vi "MainNR.vi"(10 "JQMHStartup":refnum<class "ModuleStartup.lvclass">, 11 "ErrorViewer in":refnum<class "ErrorViewer.lvclass">) -> ()   [LabVIEW 2025, in "ErrorViewer.lvclass"]
uses:
  ErrorViewer.lvclass
  C:/Git/JA/JQMH/RQMHCore/ModuleCore/Module.lvclass
  RQMHCore/Startup/ModuleStartup.lvclass
  RQMHCore/ErrorReporting/Record/LogRecord.lvclass
  RQMHCore/ModuleCore/Module.lvclass/Module.ctl
  RQMHCore/ErrorReporting/Record/LogRecord.lvclass/LogRecord.ctl
  ErrorLogBuffer/ErrorLogBuffer.lvclass/ErrorLogBuffer.ctl
  RQMHCore/ModuleCore/Reply.ctl
  RQMHCore/ActionStack/Stack/Stack.lvclass/Stack.ctl
  RQMHCore/ModuleCore/InitialiseReplyArgs.ctl
  <vilib>/Utility/miscctls.llb/LVPointTypeDef.ctl
  <vilib>/Utility/miscctls.llb/LVRowAndColumnTypeDef.ctl
  Do Something ReplyArgs.ctl
  RQMHCore/ErrorReporting/Record/Read Time.vi
  RQMHCore/ErrorReporting/Record/Read Level.vi
  RQMHCore/ErrorReporting/Record/Read Source.vi
  RQMHCore/ErrorReporting/Record/Read Message.vi
  RQMHCore/ActionStack/Stack/AppendStacks.vi
  RQMHCore/ModuleCore/Read ModuleName.vi
  RQMHCore/ErrorReporting/Record/Read Error.vi
  ErrorLogBuffer/Wrap.vi
  RQMHCore/ActionStack/Stack/StackFromSingleWithPayload.vi
  RQMHCore/ActionStack/Stack/InitFromString.vi
  RQMHCore/ActionStack/Stack/Stack.lvclass
  RQMHCore/ModuleCore/Module.lvclass
  DataStructures/src/DataTypes/Cyclic Table/Cyclic Table.lvclass
  ErrorLogBuffer/ErrorLogBuffer.lvclass
panel:
  out "Error":errorcluster
  out "error out":errorcluster
  out "Table":string[][](table)
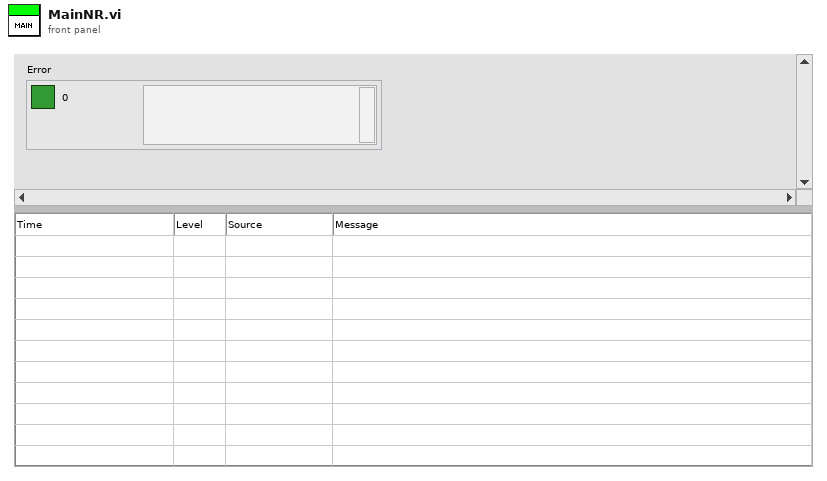
[diagram p1: front panel]
types:
  T1 = typedef "ErrorViewer.lvclass/Request Events--cluster.ctl" = cluster{"Do Something":refnum<user-event>, "Inject Log Event":refnum<user-event>}
  T2 = cluster{"StandardRequests":refnum<event-registration>, "Event Registration Refnum":refnum<event-registration>}
  T3 = cluster{"Module":refnum<class "ErrorViewer.lvclass">, "ErrorLog":refnum<class "ErrorLogBuffer.lvclass">, "Cyclic Table":refnum<class "Cyclic Table.lvclass">}
  T4 = typedef "Module.lvclass/Reply.ctl" = cluster{"Expects Reply":bool, "Reply":refnum<notifier>}
  T5 = enum32{"Invalid", "Standard", "Closed", "Hidden", "Minimized", "Maximized"}
  T6 = typedef "Module.lvclass/InitialiseReplyArgs.ctl" = cluster{"Did Init?":bool}
  T7 = typedef "LVPointTypeDef.ctl" = cluster{"Horizontal":i16, "Vertical":i16}
  T8 = typedef "LVRowAndColumnTypeDef.ctl" = cluster{"Row":i32, "Column":i32}
  T9 = typedef "ErrorViewer.lvclass/Do Something ReplyArgs.ctl" = cluster{"Value":dbl}
  T10 = typedef "JQMHModule.lvclass/Show Front Panel--Args.ctl" = variant
  T11 = typedef "JQMHModule.lvclass/Show Block Diagram.ctl" = bool
  T12 = typedef "JQMHModule.lvclass/Reply.ctl" = cluster{"Expects Reply":bool, "Reply":refnum<notifier>}
  T13 = typedef "LVPoint32TypeDef.ctl" = cluster{"Horizontal":i32, "Vertical":i32}
  T14 = typedef "LoggerShared.lvlib/Level.ctl" = enum16{"DEBUG", "INFO", "WARNING", "ERROR", "CRITICAL"}
  T15 = typedef "ErrorViewer.lvclass/Do Something Args.ctl" = cluster{"Msg":string}
  T16 = typedef "ErrorLogBuffer.lvclass/Type.ctl" = refnum<class "LogRecord.lvclass">
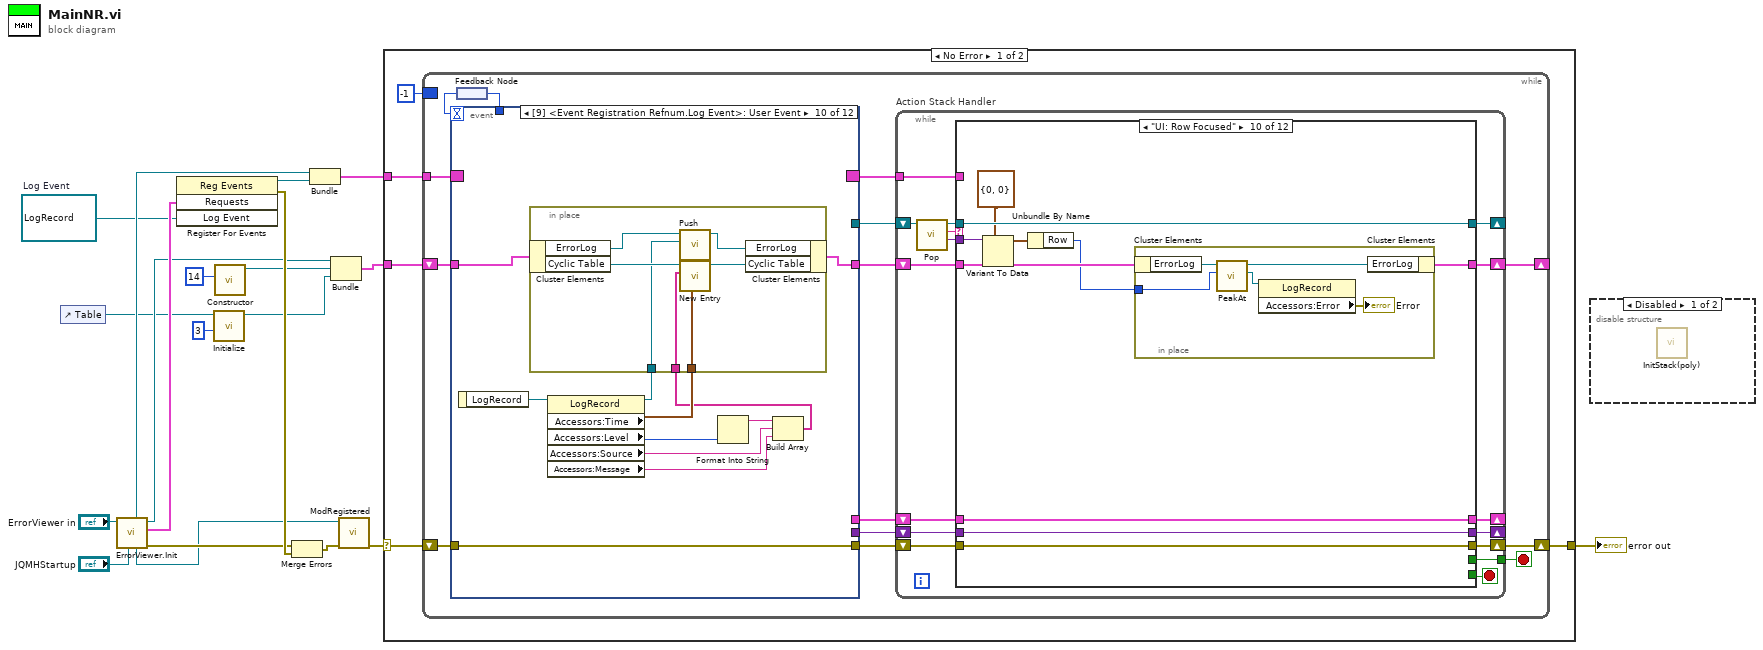
[diagram p0: block diagram]
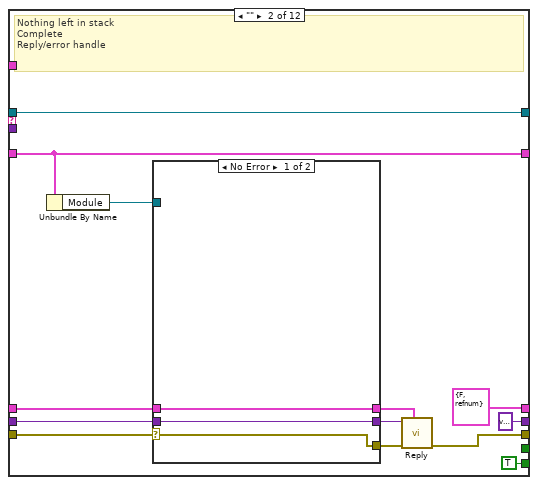
[diagram p3: hidden frame]
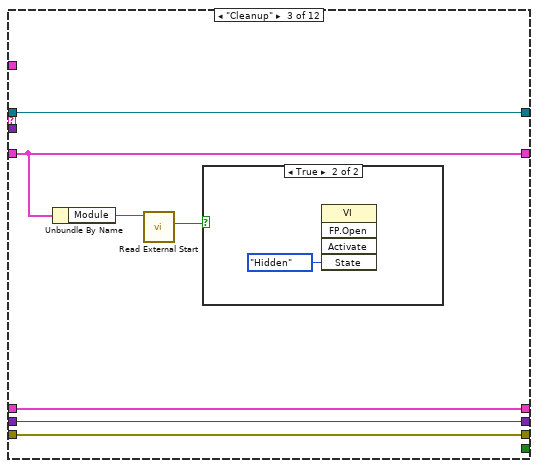
[diagram p5: hidden frame]
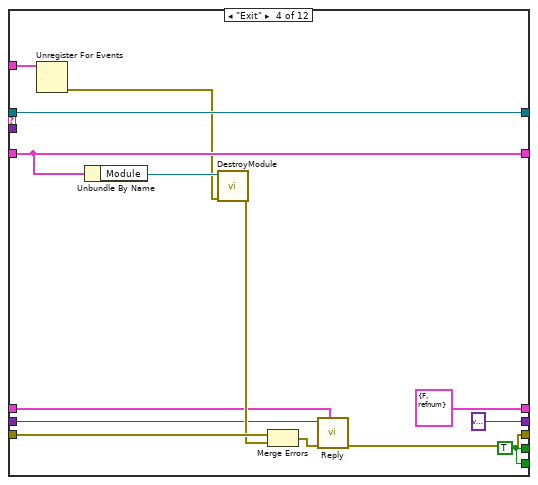
[diagram p7: hidden frame]
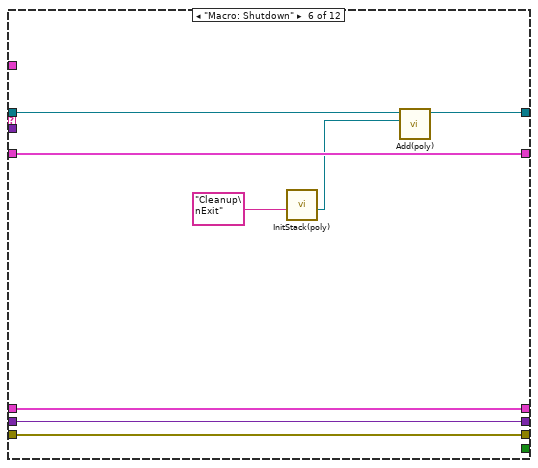
[diagram p9: hidden frame]
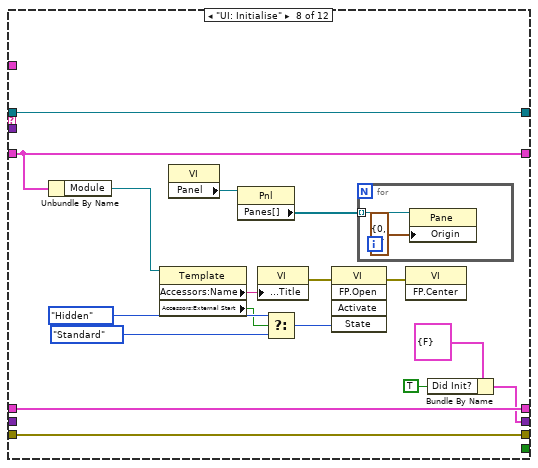
[diagram p11: hidden frame]
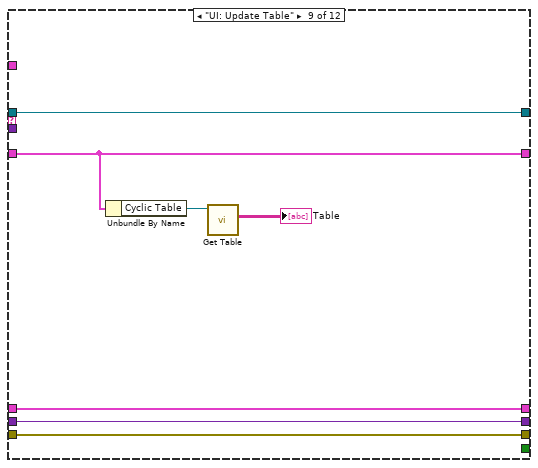
[diagram p12: hidden frame]
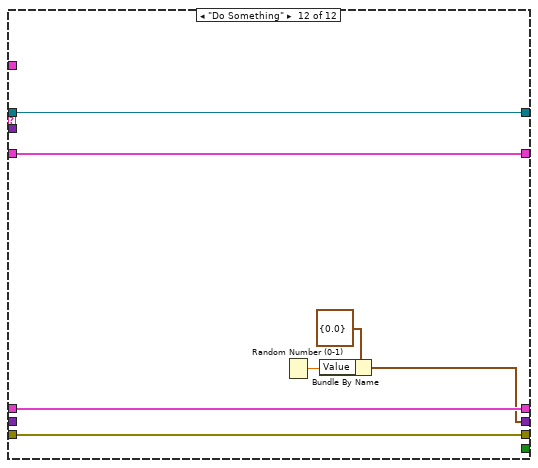
[diagram p14: hidden frame]
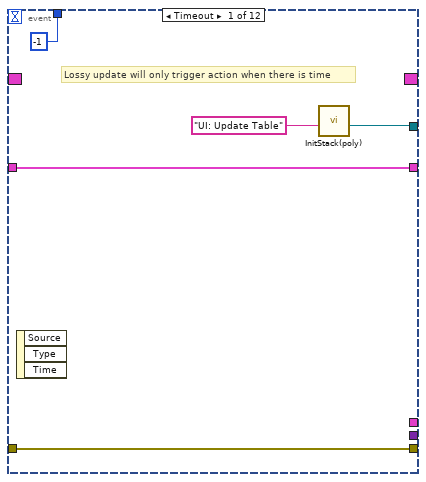
[diagram p15: hidden frame]
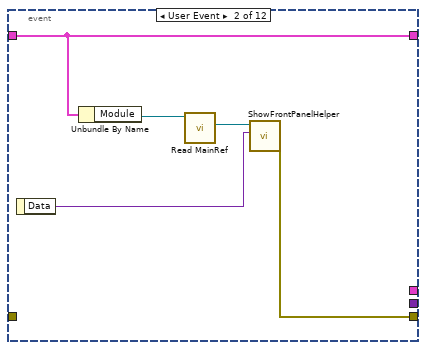
[diagram p16: hidden frame]
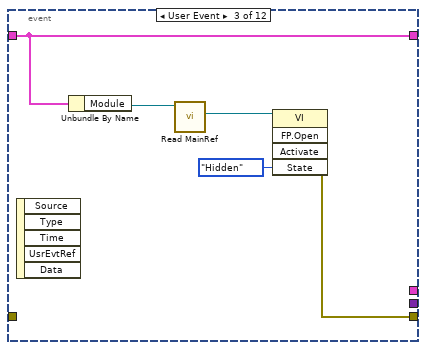
[diagram p17: hidden frame]
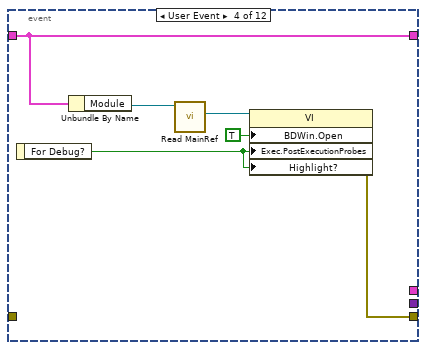
[diagram p18: hidden frame]
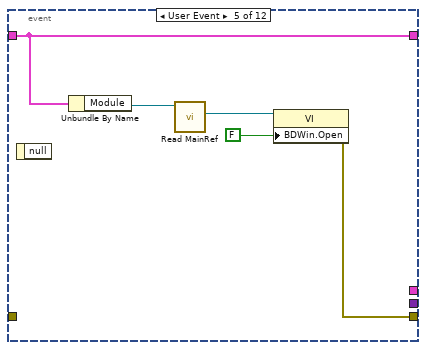
[diagram p19: hidden frame]
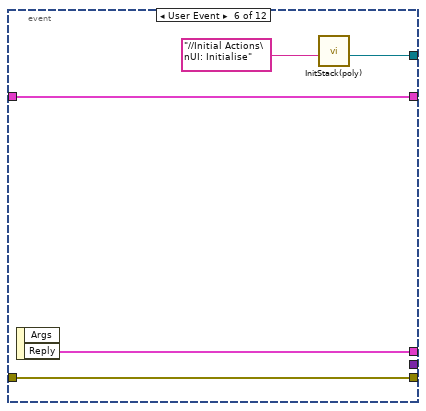
[diagram p20: hidden frame]
diagram:
  w6 = refnum<user-event> refnum  # Log Event
  n1 = control-ref of="Table"() -> (w4:refnum<vi>)
  n2 = call "ErrorViewer.Init.vi"("JQMHStartup in"="JQMHStartup", "ErrorViewer in"="ErrorViewer in") -> ("error out"=w16:errorcluster, "Requests"=w11:T1, "Module"=w8:refnum<class "ErrorViewer.lvclass">, "JQMHStartup out"=w15:refnum<class "ModuleStartup.lvclass">, "StandardRequests"=w7:refnum<event-registration>)  [unwired: 3 in, 2 out]
  n3 = register-events(w11, w6) -> (reference out=w12:refnum<event-registration>, error out=w20:errorcluster)  [unwired: 2 in]
  n4 = call "Initialize.vi"("# columns"=3, "Table"=w4) -> ("Cyclic Table"=w5:refnum<class "Cyclic Table.lvclass">)  [unwired: 8 in, 1 out]
  n5 = call "Constructor.vi"("Capacity 2^n"=u32 14 ("Capacity")) -> ("ErrorLog"=w2:refnum<class "ErrorLogBuffer.lvclass">)  [unwired: 10 in]
  n6 = Merge Errors(w16, w20) -> (w13:errorcluster)
  n7 = Bundle("StandardRequests"=w7, "Event Registration Refnum"=w12) -> (w9:T2)  [unwired: 1 in]
  n8 = Bundle("Module"=w8, "ErrorLog"=w2, "Cyclic Table"=w5) -> (w10:T3)  [unwired: 1 in]
  n9 = call "ModRegistered.vi"("error in (no error)"=w13, "JQMHStartup in"=w15) -> ("error out"=w14:errorcluster)  [unwired: 9 in]
  n10 = case "RQMH_MAIN" shown="No Error" w14 {
    selector: w14 -> [w24 w259]
    tunnel: w9 -> [w22 w258]
    tunnel: [w25 w259] -> w18
    tunnel: w10 -> [w23 w257]
    frame No Error {
      n11 = while {
        shift-right: [w32] -> w25
        shift-left: w24 -> [w39]
        shift-right: [w34] -> _
        shift-left: w23 -> [w35]
        tunnel: w22 -> [w28]
        border: -1 -> [_]
        stop <- w31 stop-if-true
        n12 = feedback #1() -> (w26:i32)
        n13 = event "RQMH_EVENT_MAIN" shown="[9] <Event Registration Refnum.Log Event>: User Event" {
          selector: w28 -> [_ _ _ _ _ _ _ _ _ _ _ w254]
          dyn-events: [_ _ _ _ _ _ _ _ _ _ _ _] -> w38
          timeout: w26 -> [_ _ _ _ _ _ _ _ _ _ _ _]
          tunnel: w39 -> [w177 _ _ _ _ w203 w208 w217 w224 w235 w248 w250]
          tunnel: [w177 w179 w183 w188 w194 w203 w208 w217 w224 w235 w248 w252] -> w33
          tunnel: [w173 _ _ _ _ w199 w204 w215 w218 _ w243 _] -> w37
          tunnel: w35 -> [w176 w182 w185 w192 w197 w202 w206 w214 w223 w233 w246 w255]
          tunnel: [w176 w182 w185 w192 w197 w202 w206 w214 w223 w234 w246 w255] -> w36
          tunnel: [_ _ _ _ _ w201 _ _ _ _ w244 w249] -> w30
          tunnel: [_ _ _ _ _ _ variant _ _ _ _ _] -> w29
          tunnel: [-1 _ _ _ _ _ _ _ _ _ _ _] -> w27
          event Timeout {
            # "Lossy update will only trigger action when there is time"
            n14 = event-data() -> ()  [unwired: 1 in, 3 out]
            n15 = call-poly "InitStack(poly).vi"("Action"="UI: Update Table") -> ("Stack out"=w173:refnum<class "Stack.lvclass">)  [unwired: 10 in]
          }
          event User Event {
            n16 = event-data() -> ("Data"=w178:T10)  [unwired: 1 in]
            n17 = Unbundle By Name(w182) -> ("Module"=w181:refnum<class "ErrorViewer.lvclass">)
            n18 = call "Read MainRef.vi"("RQMHModule in"=w181) -> ("MainRef"=w180:refnum<vi>)  [unwired: 8 in, 2 out]
            n19 = call "ShowFrontPanelHelper.vi"("Data"=w178, "VI in"=w180) -> ("error out"=w179:errorcluster)  [unwired: 9 in]
          }
          event User Event {
            n20 = event-data() -> ()  [unwired: 1 in, 5 out]
            n21 = Unbundle By Name(w185) -> ("Module"=w186:refnum<class "ErrorViewer.lvclass">)
            n22 = call "Read MainRef.vi"("RQMHModule in"=w186) -> ("MainRef"=w184:refnum<vi>)  [unwired: 8 in, 2 out]
            n23 = invoke class="VI" method="FP.Open"(reference=w184, "State"=T5."Hidden") -> (error out=w183:errorcluster)  [unwired: 3 in, 4 out]
          }
          event User Event {
            n24 = event-data() -> ("For Debug?"=w189:T11)  [unwired: 1 in]
            n25 = Unbundle By Name(w192) -> ("Module"=w193:refnum<class "ErrorViewer.lvclass">)
            n26 = call "Read MainRef.vi"("RQMHModule in"=w193) -> ("MainRef"=w190:refnum<vi>)  [unwired: 8 in, 2 out]
            n27 = property class="VI"(reference=w190, "BDWin.Open"=TRUE ("Block Diagram Window:Open"), "Exec.PostExecutionProbes"=w189, "Highlight?"=w189) -> (error out=w188:errorcluster)  [unwired: 1 in, 1 out]
          }
          event User Event {
            n28 = event-data() -> ()  [unwired: 1 in, 1 out]
            n29 = Unbundle By Name(w197) -> ("Module"=w198:refnum<class "ErrorViewer.lvclass">)
            n30 = call "Read MainRef.vi"("RQMHModule in"=w198) -> ("MainRef"=w195:refnum<vi>)  [unwired: 8 in, 2 out]
            n31 = property class="VI"(reference=w195, "BDWin.Open"=FALSE ("Block Diagram Window:Open")) -> (error out=w194:errorcluster)  [unwired: 1 in, 1 out]
          }
          event User Event {
            n32 = event-data() -> ("Reply"=w201:T12)  [unwired: 1 in, 1 out]
            n33 = call-poly "InitStack(poly).vi"("ActionStack String"="//Initial Actions\nUI: Initialise") -> ("ActionStack out"=w199:refnum<class "Stack.lvclass">)  [unwired: 10 in]
          }
          event User Event {
            (unwired) errorcluster {"status"=FALSE, "code"=0, "source"=""} ("error out")
            (unwired) TRUE
            n34 = event-data() -> ()  [unwired: 1 in, 1 out]
            n35 = call-poly "InitStack(poly).vi"("Action"="Macro: Shutdown") -> ("Stack out"=w204:refnum<class "Stack.lvclass">)  [unwired: 10 in]
          }
          event Panel Close? {
            n36 = event-data() -> ()  [unwired: 1 in, 4 out]
            n37 = Unbundle By Name(w214) -> ("Module"=w213:refnum<class "ErrorViewer.lvclass">)
            n38 = call "Read External Start.vi"("JQMHModule in"=w213) -> ("External Start?"=w212:bool)  [unwired: 8 in, 2 out]
            n39 = Select(t="", s=w212, f="Macro: Shutdown" ("Action")) -> (s? t:f=w209:string)
            n40 = call-poly "InitStack(poly).vi"("Action"=w209) -> ("Stack out"=w215:refnum<class "Stack.lvclass">)  [unwired: 10 in]
            n41 = event-data("Discard?"=TRUE) -> ()  [unwired: 1 in, 1 out]
          }
          event "Table": Mouse Down? {
            n42 = event-data() -> ("CtlRef"=w222:refnum<vi>, "Coords"=w221:T13)  [unwired: 1 in, 1 out]
            n43 = invoke class="Tbl (strict)" method="Point To Row Column"(reference=w222, "Point"=w221) -> ("CellPosition"=w219:T8)  [unwired: 4 in, 5 out]
            n44 = event-data() -> ()  [unwired: 5 in, 1 out]
            n45 = call-poly "InitStack(poly).vi"("Payload"=w219, "Action"="UI: Row Focused") -> ("Stack out"=w218:refnum<class "Stack.lvclass">)  [unwired: 9 in]
          }
          event User Event {
            n46 = event-data() -> ("LogRecord"=w232:refnum<class "LogRecord.lvclass">)  [unwired: 1 in]
            n47 = property class="LogRecord"(reference=w232) -> (reference out=w225:refnum<class "LogRecord.lvclass">, "Accessors:Time"=w231:timestamp, "Accessors:Level"=w230:T14, "Accessors:Source"=w228:string, "Accessors:Message"=w227:string)  [unwired: 1 in, 1 out]
            n48 = Format Into String(w230) -> (resulting string=w229:string)  [unwired: 3 in, 1 out]
            n49 = Build Array(w229, w228, w227) -> (w226:string[])
            n50 = in-place {
              in-place-border: w231 -> [w240]
              in-place-border: w226 -> [w239]
              in-place-border: w225 -> [w236]
              n51 = in-place-cluster #2(w233) -> ("ErrorLog"=w238:refnum<class "ErrorLogBuffer.lvclass">, "Cyclic Table"=w242:refnum<class "Cyclic Table.lvclass">)
              n52 = call "Push.vi"("Element"=w236, "POTTypedCircularBuffer in"=w238) -> ("POTTypedCircularBuffer in"=w237:refnum<class "ErrorLogBuffer.lvclass">)  [unwired: 9 in]
              n53 = call "New Entry.vi"("Time Stamp (Now)"=w240, "New Entry"=w239, "Cyclic Table in"=w242) -> ("Cyclic Table out"=w241:refnum<class "Cyclic Table.lvclass">)  [unwired: 8 in]
              n54 = in-place-cluster #2("ErrorLog"=w237, "Cyclic Table"=w241) -> (w234:T3)
            }
          }
          event User Event {
            n55 = event-data() -> ("Args"=w245:T15, "Reply Payload"=w244:T4)  [unwired: 1 in]
            n56 = call-poly "InitStack(poly).vi"("Payload"=w245, "Action"="Do Something" ("Message")) -> ("Stack out"=w243:refnum<class "Stack.lvclass">)  [unwired: 9 in]
          }
          event User Event {
            n57 = event-data() -> ("Args.Log Event"=w251:refnum<user-event>, "Reply Payload"=w249:T4)  [unwired: 1 in]
            n58 = Unbundle By Name(w254) -> ("Event Registration Refnum"=w253:refnum<event-registration>)
            n59 = register-events(reference=w253, error in=w250, w251) -> (error out=w252:errorcluster)  [unwired: 1 in, 1 out]
          }
        }
        n60 = feedback-in #1(w27) -> ()
        n61 = while "Action Stack Handler" {
          shift-right: [w55] -> _
          shift-left: w37 -> [w47]
          shift-right: [w52] -> w32
          shift-left: w33 -> [w53]
          tunnel: w38 -> [w51]
          shift-right: [w49] -> w34
          shift-left: w36 -> [w50]
          tunnel: [w48] -> w31
          shift-right: [w42] -> _
          shift-left: w30 -> [w43]
          shift-right: [w41] -> _
          shift-left: w29 -> [w40]
          stop <- w54 stop-if-true
          n62 = call "Pop.vi"("Stack in"=w47) -> ("Popped Payload"=w44:variant, "Popped Action"=w45:string, "Stack out"=w46:refnum<class "Stack.lvclass">)  [unwired: 8 in]
          n63 = case shown="\"UI: Row Focused\"" w45 {
            tunnel: w46 -> [w60 w73 w86 w101 w106 w109 w119 w136 w145 w155 w165 w172]
            tunnel: [w60 w73 w86 w101 w106 w107 w119 w136 w145 w155 w165 w172] -> w55
            tunnel: w44 -> [_ _ _ _ _ _ _ _ _ w151 _ _]
            tunnel: [_ TRUE ("Boolean") _ w99 _ _ _ _ _ _ _ _] -> w54
            tunnel: w53 -> [w56 w71 w85 w93 w104 w113 w118 w135 w144 w154 w164 w171]
            tunnel: [w56 w66 w85 w88 w104 w113 w118 w135 w144 w154 w164 w171] -> w52
            tunnel: w51 -> [_ _ _ w100 _ _ _ _ _ _ _ _]
            tunnel: w50 -> [w59 w70 w81 w95 w105 w114 w117 w128 w141 w148 w163 w170]
            tunnel: [w59 w70 w81 w95 w105 w114 w117 w128 w141 w146 w163 w170] -> w49
            tunnel: [_ _ _ w99 _ _ _ _ _ _ _ _] -> w48
            tunnel: w43 -> [w58 w67 w84 w89 w103 w112 w116 w134 w143 w153 w162 w169]
            tunnel: [w58 T4 {"Expects Reply"=FALSE, "Reply"=refnum} ("Reply Payload") w84 T4 {"Expects Reply"=FALSE, "Reply"=refnum} ("Reply Payload") w103 w112 w116 w134 w143 w153 w162 w169] -> w42
            tunnel: [w57 variant ("Variant") w83 variant ("Variant") w102 w111 w115 w120 w142 w152 w161 w166] -> w41
            tunnel: w40 -> [w57 w62 w83 w90 w102 w111 w115 _ w142 w152 w161 _]
            frame Default {
              # "#TODO Add Error Handling"
            }
            frame "" {
              # "Nothing left in stack\nComplete\nReply/error handle"
              n64 = Unbundle By Name(w70) -> ("Module"=w69:refnum<class "ErrorViewer.lvclass">)
              n65 = case shown="No Error" w71 {
                selector: w71 -> [w74 w78]
                tunnel: [w76 w79] -> w68
                tunnel: w67 -> [w76 w79]
                tunnel: [w75 w77] -> w63
                tunnel: w62 -> [w75 w77]
                tunnel: w69 -> [_ _]
                tunnel: [w74 w78] -> w61
                frame No Error {
                }
                frame Error {
                }
              }
              n66 = call "Reply.vi"("Reply"=w68, "error in (no error)"=w61, "ReplyPayload"=w63) -> ("error out"=w66:errorcluster)  [unwired: 8 in]
            }
            frame "Cleanup" {
              n67 = Unbundle By Name(w81) -> ("Module"=w82:refnum<class "ErrorViewer.lvclass">)
              n68 = call "Read External Start.vi"("JQMHModule in"=w82) -> ("External Start?"=w80:bool)  [unwired: 8 in, 2 out]
              n69 = case shown="True" w80 {
                frame False {
                }
                frame True {
                  n70 = invoke class="VI" method="FP.Open"("State"=T5."Hidden") -> ()  [unwired: 4 in, 5 out]
                }
              }
            }
            frame "Exit" {
              w99 = TRUE
              n71 = Unregister For Events(event registration refnum=w100) -> (error out=w94:errorcluster)  [unwired: 1 in]
              n72 = Unbundle By Name(w95) -> ("Module"=w96:refnum<class "ErrorViewer.lvclass">)
              n73 = call "DestroyModule.vi"("error in (no error)"=w94, "JQMHModule in"=w96) -> ("error out"=w92:errorcluster)  [unwired: 9 in]
              n74 = Merge Errors(w93, w92) -> (w91:errorcluster)
              n75 = call "Reply.vi"("Reply"=w89, "error in (no error)"=w91, "ReplyPayload"=w90) -> ("error out"=w88:errorcluster)  [unwired: 8 in]
            }
            frame "---------- Macros ----------" {
            }
            frame "Macro: Shutdown" {
              n76 = call-poly "InitStack(poly).vi"("ActionStack String"="Cleanup\nExit") -> ("ActionStack out"=w108:refnum<class "Stack.lvclass">)  [unwired: 10 in]
              n77 = call-poly "Add(poly).vi"("Second"=w108, "First"=w109) -> ("First"=w107:refnum<class "Stack.lvclass">)  [unwired: 9 in]
            }
            frame "---------- UI ----------" {
              # "Add module specific commands"
            }
            frame "UI: Initialise" {
              n78 = Unbundle By Name(w128) -> ("Module"=w127:refnum<class "ErrorViewer.lvclass">)
              n79 = property class="Template"(reference=w127) -> ("Accessors:Name"=w126:string, "Accessors:External Start"=w124:bool)  [unwired: 1 in, 2 out]
              n80 = property on="Property Node" class="VI"() -> ("Panel"=w130:refnum<vi>)  [unwired: 2 in, 2 out]
              n81 = property on="Property Node" class="Pnl"(reference=w130) -> ("Panes[]"=w129:refnum<vi>[])  [unwired: 1 in, 2 out]
              n82 = property on="Property Node" class="VI"("Front Panel.Title"=w126) -> (error out=w133:errorcluster)  [unwired: 2 in, 1 out]
              n83 = Select(t=T5."Hidden" ("State"), s=w124, f=T5."Standard" ("State")) -> (s? t:f=w123:T5)
              n84 = invoke on="Invoke Node" class="VI" method="FP.Open"(error in=w133, "State"=w123) -> (error out=w132:errorcluster)  [unwired: 3 in, 4 out]
              n85 = for {
                tunnel: w129 -> [w137] mode=indexing
                n86 = property on="Property Node" class="Pane"(reference=w137, "Origin"=T7 {"Horizontal"=0, "Vertical"=0}) -> ()  [unwired: 1 in, 2 out]
              }
              n87 = invoke on="Invoke Node" class="VI" method="FP.Center"(error in=w132) -> ()  [unwired: 2 in, 3 out]
              n88 = Bundle By Name(cluster=T6 {"Did Init?"=FALSE} ("Args"), "Did Init?"=TRUE) -> (w120:T6)
            }
            frame "UI: Update Table" {
              n89 = Unbundle By Name(w141) -> ("Cyclic Table"=w140:refnum<class "Cyclic Table.lvclass">)
              n90 = call "Get Table.vi"("Cyclic Table in"=w140) -> ("Table Data (sorted by time)"=→"Table":string[][])  [unwired: 10 in]
            }
            frame "UI: Row Focused" {
              n91 = Variant To Data(type=T8 {"Row"=0, "Column"=0} ("Cell Position"), Variant=w151) -> (data=w149:T8)  [unwired: 1 in, 1 out]
              n92 = Unbundle By Name(w149) -> ("Row"=w147:i32)
              n93 = in-place {
                in-place-border: w147 -> [w156]
                n94 = in-place-cluster #3(w148) -> ("ErrorLog"=w160:refnum<class "ErrorLogBuffer.lvclass">)
                n95 = call "PeakAt.vi"("Index"=w156, "POTTypedCircularBuffer in"=w160) -> ("element"=w158:T16, "POTTypedCircularBuffer out"=w159:refnum<class "ErrorLogBuffer.lvclass">)  [unwired: 8 in]
                n96 = property class="LogRecord"(reference=w158) -> ("Accessors:Error"=→"Error":errorcluster)  [unwired: 1 in, 2 out]
                n97 = in-place-cluster #3("ErrorLog"=w159) -> (w146:T3)
              }
            }
            frame "---------- Actions ----------" {
              # "Add module specific commands"
            }
            frame "Do Something" {
              n98 = Random Number (0-1)() -> (number: 0 to 1=w168:dbl)
              n99 = Bundle By Name(cluster=T9 {"Value"=0.0} ("ReplyArgs"), "Value"=w168) -> (w166:T9)
            }
          }
        }
      }
    }
    frame Error {
      n100 = Unregister For Events(event registration refnum=w258) -> ()  [unwired: 1 in, 1 out]
      n101 = Unbundle(w257) -> ("Module"=w256:refnum<class "ErrorViewer.lvclass">)  [unwired: 2 out]
      n102 = call "DestroyModule.vi"("JQMHModule in"=w256) -> ()  [unwired: 10 in, 1 out]
    }
  }
  "error out" <- w18
  n103 = disable-structure shown="Disabled" {
    frame Disabled {
      n104 = call-poly "InitStack(poly).vi"() -> ()  [unwired: 11 in, 1 out]
    }
    frame Enabled {
    }
  }
